vi "Class Tree_Select first or last item.vi"(7 "Select Item":enum16{"First", "Last"}(ring), 8 "error in (no error)":errorcluster, 11 "Tree Ref":refnum<vi>) -> (0 "error out":errorcluster)   [LabVIEW 2023]
doc: "If last and down, go to first; if first and up, go to last."
panel:
  in  "Tree":string[](tree)
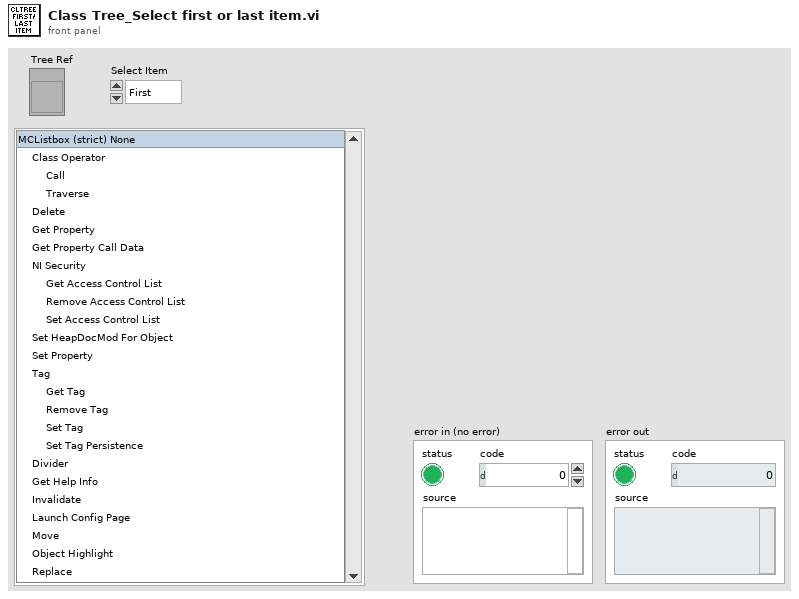
[diagram p1: front panel]
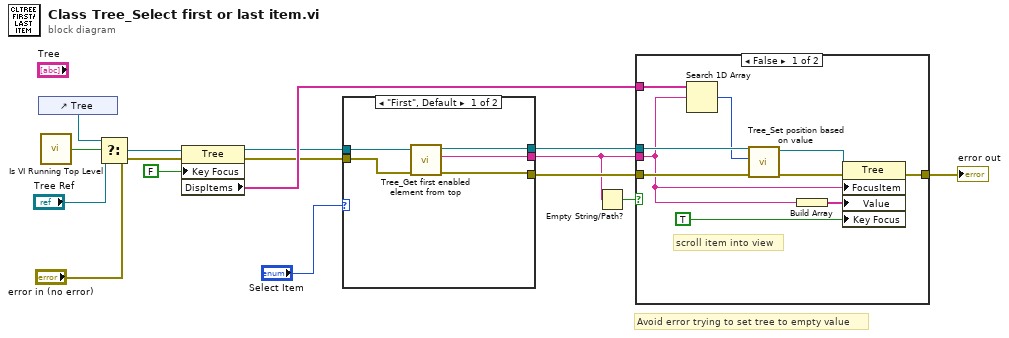
[diagram p0: block diagram]
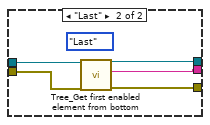
[diagram p3: hidden frame]
diagram:
  # "Avoid error trying to set tree to empty value"
  n1 = control-ref of="Tree"() -> (w14:refnum<vi>)
  n2 = call "Is VI Running Top Level.vi"() -> ("Top Level?"=w15:bool)  [unwired: 5 in]
  n3 = Select(t=w14, s=w15, f="Tree Ref") -> (s? t:f=w13:refnum<vi>)
  n4 = property class="Tree"(reference=w13, error in="error in (no error)", "Key Focus"=FALSE) -> (reference out=w6:refnum<vi>, error out=w4:errorcluster, "DispItems"=w8:string[])
  n5 = case shown="\"First\", Default" "Select Item" {
    tunnel: w6 -> [w20 w25]
    tunnel: [w19 w24] -> w5
    tunnel: [w18 w23] -> w2
    tunnel: w4 -> [w17 w22]
    tunnel: [w16 w21] -> w3
    frame "First", Default {
      n6 = call "Tree_Get first enabled element from top.vi"("error in (no error)"=w17, "Tree Control Ref"=w20) -> ("error out"=w16:errorcluster, "First Enabled Element"=w18:string, "Tree Control Ref Out"=w19:refnum<vi>)  [unwired: 7 in]
    }
    frame "Last" {
      (unwired) enum16{"First", "Last"}."Last" ("Select Item")
      n7 = call "Tree_Get first enabled element from bottom.vi"("error in (no error)"=w22, "TreeControl Ref"=w25) -> ("error out"=w21:errorcluster, "First Element Tag"=w23:string, "Tree Control Ref Out"=w24:refnum<vi>)  [unwired: 7 in]
    }
  }
  n8 = Empty String/Path?(string/path=w2) -> (empty?=w1:bool)
  n9 = case shown="False" w1 {
    tunnel: [w35 w36] -> w10
    tunnel: w8 -> [w34 _]
    tunnel: w5 -> [w33 _]
    tunnel: w3 -> [w32 w36]
    tunnel: w2 -> [w31 _]
    frame False {
      # "scroll item into view"
      n10 = Search 1D Array(1D array=w34, element=w31) -> (index of element=w28:i32)  [unwired: 1 in]
      n11 = call "Tree_Set position based on value.vi"("error in (no error)"=w32, "Selected Row"=w28, "Tree Ref"=w33) -> ("error out"=w27:errorcluster, "Tree Ref"=w29:refnum<vi>)  [unwired: 7 in]
      n12 = Build Array(w31) -> (w26:string[])
      n13 = property class="Tree"(reference=w29, error in=w27, "FocusItem"=w31, "Value"=w26, "Key Focus"=TRUE) -> (error out=w35:errorcluster)  [unwired: 1 out]
    }
    frame True {
    }
  }
  "error out" <- w10
